vi "BPM-Chassis02 FPGA.vi"() -> ()   [LabVIEW 2011]
uses:
  <vilib>/rvi/eio/common/nirviEmuTemplateMethod_errors.vi
  <vilib>/eio/EIONode/EIONode.xnode
  <vilib>/eio/EIOMethodNode/EIOMethodNode.xnode
panel:
  out "Timestamp":u32 caption="Tick Count(Ticks)"
  out "Mod1/AI0":fxp<+/-,20,5> format="%.17g"
  out "Mod1/AI2":fxp<+/-,20,5> format="%.17g"
  out "Mod1/AI3":fxp<+/-,20,5> format="%.17g"
  out "Mod2/AI0":fxp<+/-,20,5> format="%.17g"
  out "Mod2/AI1":fxp<+/-,20,5> format="%.17g"
  out "Mod2/AI2":fxp<+/-,20,5> format="%.17g"
  out "Mod2/AI3":fxp<+/-,20,5> format="%.17g"
  out "Mod1/AI1":fxp<+/-,20,5> format="%.17g"
  out "period":u32
  out "delay":u32
  out "dperiod":u32
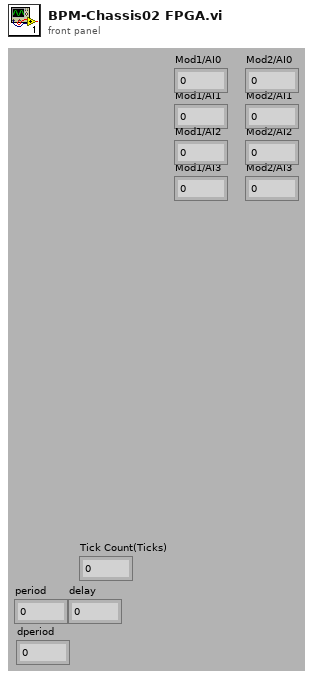
[diagram p1: front panel]
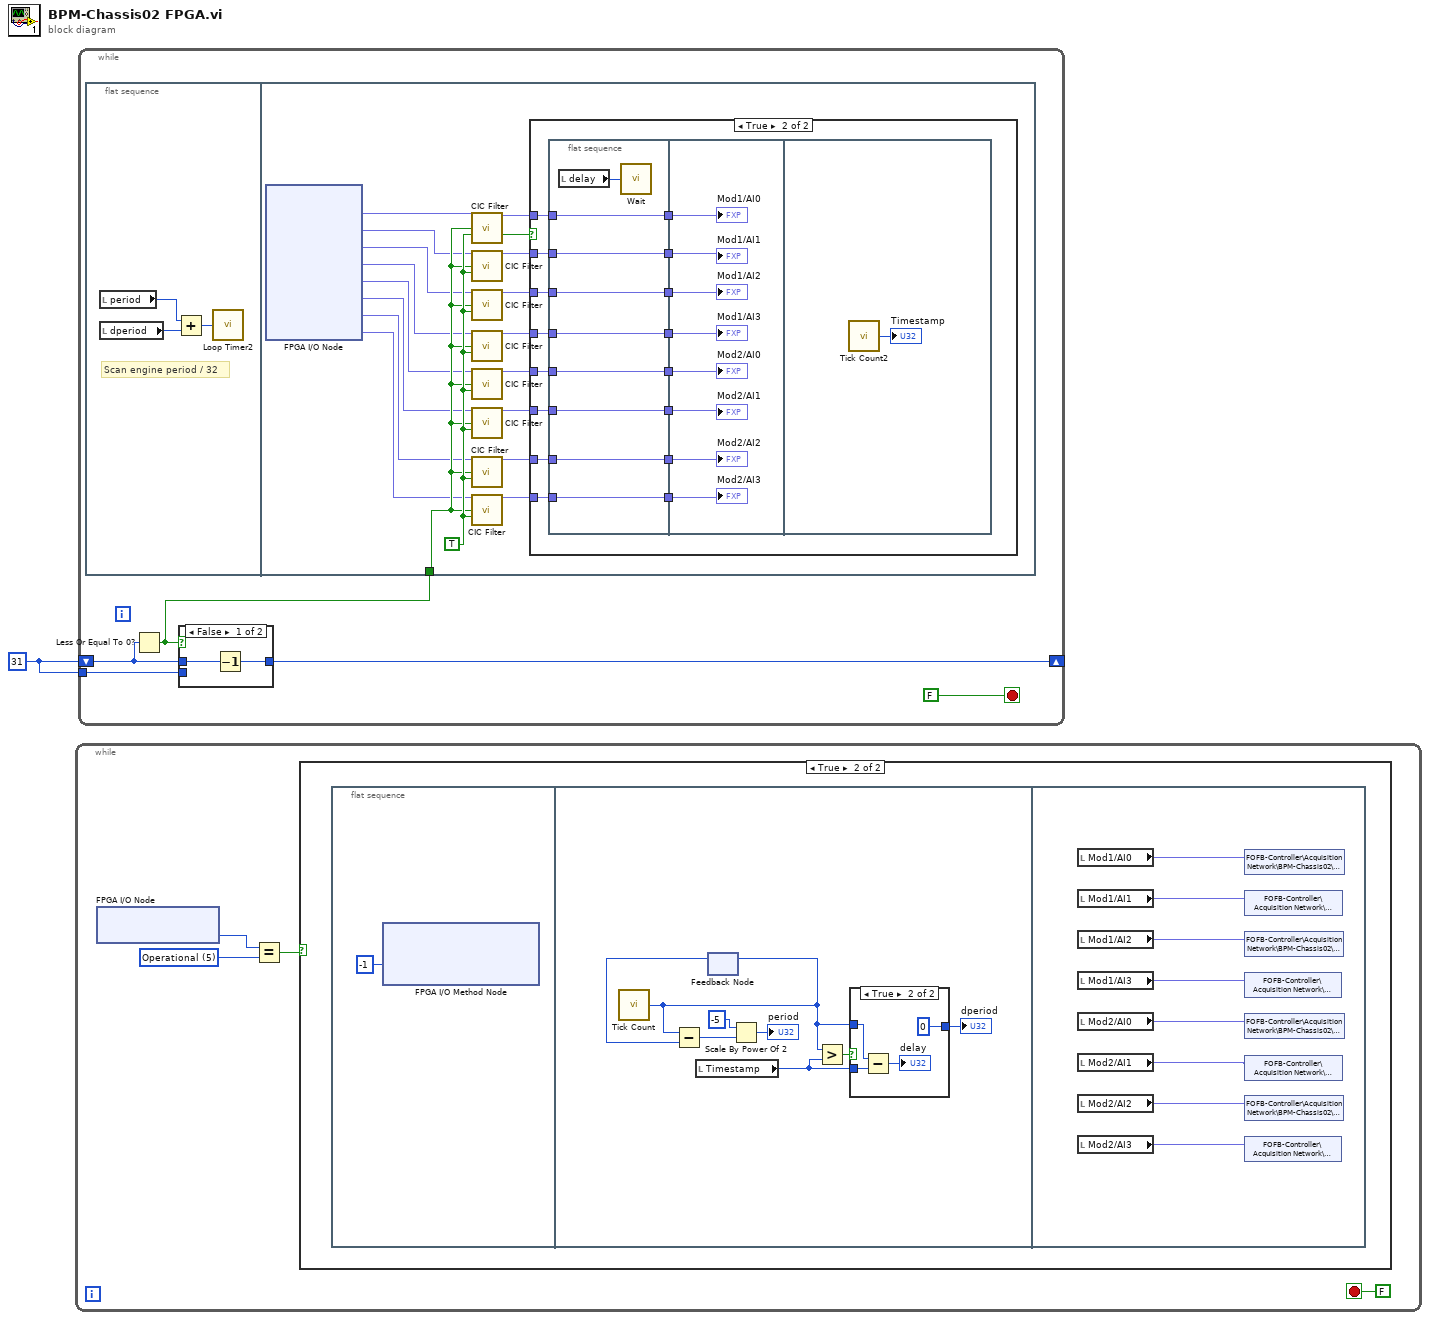
[diagram p0: block diagram]
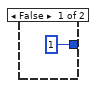
[diagram p5: hidden frame]
diagram:
  w1 = 31
  n1 = while {
    stop <- FALSE stop-if-true
    w4 = u8 5 items=["Init"=1, "PreOp"=2, "Bootstrap"=3, "SafeOp"=4, "Operational"=5]
    n2 = xnode "FPGA I/O Node"() -> ("EtherCAT State"=w3:u8)  [unwired: 1 in, 1 out]
    n3 = Equal?(x=w3, y=w4) -> (x = y?=w2:bool)
    n4 = case shown="True" w2 {
      frame False {
      }
      frame True {
        n5 = flat-sequence {
          frame #0 {
            n6 = xnode "FPGA I/O Method Node"("Timeout"=-1) -> ()  [unwired: 1 in, 2 out]
          }
          frame #1 {
            n7 = call "Tick Count"() -> ("Tick Count(Ticks)"=w8:u32)
            n8 = local read "Timestamp"() -> (w10:u32)
            n9 = feedback #1() -> (w7:u32)  [unwired: 1 in]
            n10 = Subtract(x=w8, y=w7) -> (x-y=w13:u32)
            n11 = feedback-in #1(w8) -> ()
            n12 = Scale By Power Of 2(n=i8 -5, x=w13) -> (x*2^n=→"period":u32)
            n13 = Greater?(x=w8, y=w10) -> (0:w11:bool)
            n14 = case shown="True" w11 {
              tunnel: w8 -> [_ w19]
              tunnel: w10 -> [_ w18]
              tunnel: [u32 1 ("dt 2") u32 0 ("dt 2")] -> w9
              frame False {
              }
              frame True {
                n15 = Subtract(x=w19, y=w18) -> (x-y=→"delay":u32)
              }
            }
            "dperiod" <- w9
          }
          frame #2 {
            n16 = local read "Mod1/AI0"() -> (w27:fxp<+/-,20,5>)
            n17 = local read "Mod1/AI1"() -> (w26:fxp<+/-,20,5>)
            n18 = local read "Mod1/AI2"() -> (w25:fxp<+/-,20,5>)
            n19 = local read "Mod1/AI3"() -> (w24:fxp<+/-,20,5>)
            n20 = local read "Mod2/AI0"() -> (w23:fxp<+/-,20,5>)
            n21 = local read "Mod2/AI1"() -> (w22:fxp<+/-,20,5>)
            n22 = local read "Mod2/AI2"() -> (w21:fxp<+/-,20,5>)
            n23 = local read "Mod2/AI3"() -> (w20:fxp<+/-,20,5>)
            n24 = shared-variable "FOFB-Controller\\Acquisition Network\\BPM-Chassis02\\User-Defined Variables\\AMP04AH"(w27) -> ()  [unwired: 1 in, 1 out]
            n25 = shared-variable "FOFB-Controller\\Acquisition Network\\BPM-Chassis02\\User-Defined Variables\\AMP04AV"(w26) -> ()  [unwired: 1 in, 1 out]
            n26 = shared-variable "FOFB-Controller\\Acquisition Network\\BPM-Chassis02\\User-Defined Variables\\AMP04BH"(w25) -> ()  [unwired: 1 in, 1 out]
            n27 = shared-variable "FOFB-Controller\\Acquisition Network\\BPM-Chassis02\\User-Defined Variables\\AMP04BV"(w24) -> ()  [unwired: 1 in, 1 out]
            n28 = shared-variable "FOFB-Controller\\Acquisition Network\\BPM-Chassis02\\User-Defined Variables\\AMP05AH"(w23) -> ()  [unwired: 1 in, 1 out]
            n29 = shared-variable "FOFB-Controller\\Acquisition Network\\BPM-Chassis02\\User-Defined Variables\\AMP05AV"(w22) -> ()  [unwired: 1 in, 1 out]
            n30 = shared-variable "FOFB-Controller\\Acquisition Network\\BPM-Chassis02\\User-Defined Variables\\AMP05BH"(w21) -> ()  [unwired: 1 in, 1 out]
            n31 = shared-variable "FOFB-Controller\\Acquisition Network\\BPM-Chassis02\\User-Defined Variables\\AMP05BV"(w20) -> ()  [unwired: 1 in, 1 out]
          }
        }
      }
    }
  }
  n32 = while {
    shift-right: [w31] -> _
    shift-left: w1 -> [w30]
    tunnel: w1 -> [w28]
    stop <- FALSE stop-if-true
    n33 = flat-sequence {
      tunnel: w29 -> [w54]
      frame #0 {
        # "Scan engine period / 32"
        n34 = local read "period"() -> (w38:u32)
        n35 = local read "dperiod"() -> (w37:u32)
        n36 = Add(x=w38, y=w37) -> (x+y=w36:u32)
        n37 = call "Loop Timer2"("Count(Ticks)"=w36) -> ()  [unwired: 1 out]
      }
      frame #1 {
        w55 = TRUE ("input valid")
        n38 = xnode "FPGA I/O Node"() -> ("Mod1/AI0"=w46:fxp<+/-,20,5>, "Mod1/AI1"=w45:fxp<+/-,20,5>, "Mod1/AI2"=w44:fxp<+/-,20,5>, "Mod1/AI3"=w43:fxp<+/-,20,5>, "Mod2/AI0"=w42:fxp<+/-,20,5>, "Mod2/AI1"=w41:fxp<+/-,20,5>, "Mod2/AI2"=w40:fxp<+/-,20,5>, "Mod2/AI3"=w39:fxp<+/-,20,5>)  [unwired: 8 in, 8 out]
        n39 = call "CIC Filter.vi"("input data"=w46, "sample"=w54, "input valid"=w55) -> ("output data"=w56:fxp<+/-,20,5>, "output valid"=w57:bool)  [unwired: 10 in, 1 out]
        n40 = call "CIC Filter.vi"("input data"=w45, "sample"=w54, "input valid"=w55) -> ("output data"=w53:fxp<+/-,20,5>)  [unwired: 10 in, 2 out]
        n41 = call "CIC Filter.vi"("input data"=w44, "sample"=w54, "input valid"=w55) -> ("output data"=w52:fxp<+/-,20,5>)  [unwired: 10 in, 2 out]
        n42 = call "CIC Filter.vi"("input data"=w43, "sample"=w54, "input valid"=w55) -> ("output data"=w51:fxp<+/-,20,5>)  [unwired: 10 in, 2 out]
        n43 = call "CIC Filter.vi"("input data"=w42, "sample"=w54, "input valid"=w55) -> ("output data"=w50:fxp<+/-,20,5>)  [unwired: 10 in, 2 out]
        n44 = call "CIC Filter.vi"("input data"=w41, "sample"=w54, "input valid"=w55) -> ("output data"=w49:fxp<+/-,20,5>)  [unwired: 10 in, 2 out]
        n45 = call "CIC Filter.vi"("input data"=w40, "sample"=w54, "input valid"=w55) -> ("output data"=w48:fxp<+/-,20,5>)  [unwired: 10 in, 2 out]
        n46 = call "CIC Filter.vi"("input data"=w39, "sample"=w54, "input valid"=w55) -> ("output data"=w47:fxp<+/-,20,5>)  [unwired: 10 in, 2 out]
        n47 = case shown="True" w57 {
          tunnel: w56 -> [_ w73]
          tunnel: w53 -> [_ w71]
          tunnel: w52 -> [_ w69]
          tunnel: w51 -> [_ w68]
          tunnel: w50 -> [_ w65]
          tunnel: w49 -> [_ w63]
          tunnel: w48 -> [_ w61]
          tunnel: w47 -> [_ w59]
          frame False {
          }
          frame True {
            n48 = flat-sequence {
              tunnel: w73 -> [w82]
              tunnel: [w82] -> w72
              tunnel: w71 -> [w80]
              tunnel: [w80] -> w70
              tunnel: w69 -> [w78]
              tunnel: w68 -> [w79]
              tunnel: [w79] -> w67
              tunnel: [w78] -> w66
              tunnel: w65 -> [w77]
              tunnel: [w77] -> w64
              tunnel: w63 -> [w76]
              tunnel: [w76] -> w62
              tunnel: w61 -> [w75]
              tunnel: [w75] -> w60
              tunnel: w59 -> [w74]
              tunnel: [w74] -> w58
              tunnel: w72 -> [w89]
              tunnel: w70 -> [w90]
              tunnel: w67 -> [w88]
              tunnel: w66 -> [w87]
              tunnel: w64 -> [w86]
              tunnel: w62 -> [w85]
              tunnel: w60 -> [w84]
              tunnel: w58 -> [w83]
              frame #0 {
                n49 = local read "delay"() -> (w81:u32)
                n50 = call "Wait"("Count(Ticks)"=w81) -> ()  [unwired: 1 out]
              }
              frame #1 {
                "Mod1/AI0" <- w89
                "Mod1/AI2" <- w87
                "Mod1/AI3" <- w88
                "Mod2/AI0" <- w86
                "Mod2/AI1" <- w85
                "Mod2/AI2" <- w84
                "Mod2/AI3" <- w83
                "Mod1/AI1" <- w90
              }
              frame #2 {
                n51 = call "Tick Count2"() -> ("Tick Count(Ticks)"=→"Timestamp":u32)
              }
            }
          }
        }
      }
    }
    n52 = Less Or Equal To 0?(x=w30) -> (x <= 0?=w29:bool)
    n53 = case shown="False" w29 {
      tunnel: [w34 w35] -> w31
      tunnel: w30 -> [w33 _]
      tunnel: w28 -> [_ w35]
      frame False {
        n54 = Decrement(x=w33) -> (x-1=w34:i32)
      }
      frame True {
      }
    }
  }
